vi "Translator.File.ReadGui.vi"(6 "~Do not save font? (F)":bool, 8 "~error in":errorcluster, 10 "~Language in use":string="English", 11 "~Translation folder":path=path "D:/PL_0125_Sapphire_Automation_branches/SOFTWARE_v1.1-Translation/settings") -> (0 "~error out":errorcluster, 1 "~restart?":bool, 2 "~font name":string)   [LabVIEW 2013]
uses:
  <vilib>/Utility/miscctls.llb/LVBoundsTypeDef.ctl
  Translator.Global.vi
  Config/Config.Global.vi
panel:
  out "~progressbar2":i32(slide) scale=-1.1..10.0
  out "~progressbar1":i32(slide) scale=0.0..17.0
  out "Message":string
  out "~flag":picture
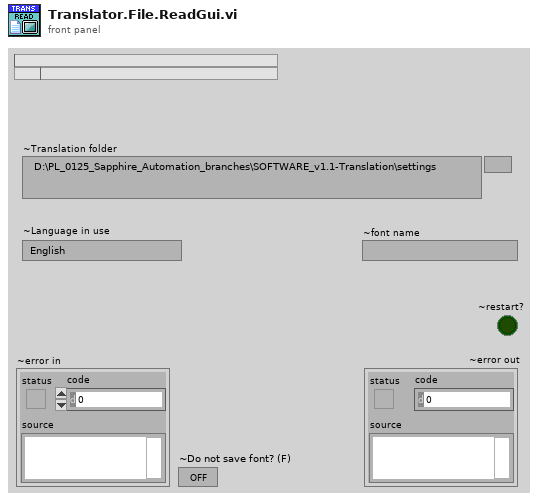
[diagram p1: front panel]
types:
  T1 = typedef "LVBoundsTypeDef.ctl" = cluster{"Width":u32, "Height":u32}
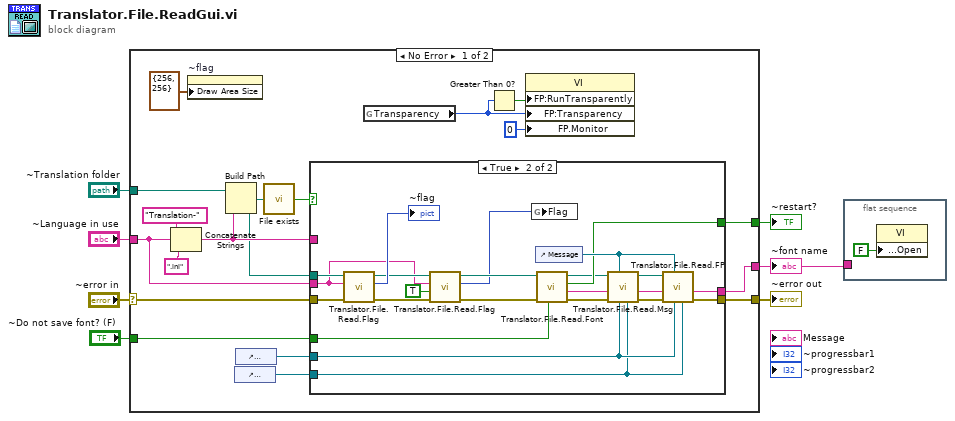
[diagram p0: block diagram]
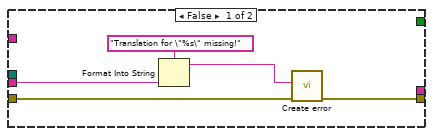
[diagram p2: hidden frame]
diagram:
  n1 = case shown="No Error" "~error in" {
    selector: "~error in" -> [w16 w48]
    tunnel: "~Translation folder" -> [w11 _]
    tunnel: [w23 w48] -> w4
    tunnel: "~Language in use" -> [w15 _]
    tunnel: [w13 _] -> w3
    tunnel: [w18 _] -> w2
    tunnel: "~Do not save font? (F)" -> [w12 _]
    frame No Error {
      n2 = Concatenate Strings("Translation-" ("string"), w15, ".ini" ("string")) -> (w22:string)
      n3 = property on="~flag" class="Pict"("Draw Area Size"=T1 {"Width"=256, "Height"=256}) -> ()  [unwired: 2 in, 2 out]
      n4 = Build Path(base path=w11, name or relative path=w22) -> (appended path=w17:path)
      n5 = control-ref of="~progressbar2"() -> (w19:refnum<vi>)
      n6 = control-ref of="~progressbar1"() -> (w20:refnum<vi>)
      n7 = call "File exists.vi"("file path"=w17) -> ("exists?"=w21:bool)  [unwired: 4 in]
      n8 = case shown="True" w21 {
        tunnel: w16 -> [w29 w39]
        tunnel: [_ w47] -> w13
        tunnel: [w30 w46] -> w23
        tunnel: w17 -> [_ w37]
        tunnel: w22 -> [_ _]
        tunnel: w20 -> [_ w45]
        tunnel: w19 -> [_ w44]
        tunnel: [_ w42] -> w18
        tunnel: w15 -> [w26 w34]
        tunnel: w12 -> [_ w31]
        frame False {
          n9 = Format Into String(format string="Translation for \"%s\" missing!", w26) -> (resulting string=w27:string)  [unwired: 2 in, 1 out]
          n10 = call "Create error.vi"("error in"=w29, "explanation"=w27) -> ("error out"=w30:errorcluster)  [unwired: 9 in]
        }
        frame True {
          n11 = call "Translator.File.Read.Flag.vi"("error in"=w39, "Language in use"=w34, "Translation file"=w37) -> ("error out"=w36:errorcluster, "~flag"=→"~flag":picture)  [unwired: 6 in, 1 out]
          n12 = call "Translator.File.Read.Flag.vi"("error in"=w36, "miniature (F)"=TRUE, "Language in use"=w34, "Translation file"=w37) -> ("error out"=w35:errorcluster, "~flag"=w32:picture)  [unwired: 5 in, 1 out]
          n13 = global write "Translator.Global.vi" "Flag"(w32) -> ()
          n14 = control-ref of="Message"() -> (w43:refnum<vi>)
          n15 = call "Translator.File.Read.Font.vi"("Do not save font? (F)"=w31, "error in"=w35, "Translation file"=w37) -> ("error out"=w41:errorcluster, "font name"=w47:string, "restart required?"=w42:bool)  [unwired: 6 in]
          n16 = call "Translator.File.Read.Msg.vi"("progressbar2"=w44, "progressbar1"=w45, "Message"=w43, "error in"=w41, "Translation folder"=w37) -> ("error out"=w40:errorcluster)  [unwired: 6 in]
          n17 = call "Translator.File.Read.FP.vi"("progressbar2"=w44, "progressbar1"=w45, "Message"=w43, "error in"=w40, "font name"=w47, "Translation file"=w37) -> ("error out"=w46:errorcluster)  [unwired: 5 in]
        }
      }
      n18 = global read "Config.Global.vi" "Transparency"() -> (w8:u8)
      n19 = Greater Than 0?(x=w8) -> (x > 0?=w10:bool)
      n20 = property class="VI"("FP:RunTransparently"=w10, "FP:Transparency"=w8, "FP.Monitor"=u16 0 ("Front Panel Window:Monitor")) -> ()  [unwired: 2 in, 2 out]
    }
    frame Error {
    }
  }
  "~error out" <- w4
  "~font name" <- w3
  "~restart?" <- w2
  n21 = flat-sequence {
    tunnel: w3 -> [_]
    frame #0 {
      n22 = property class="VI"("Front Panel.Open"=FALSE ("Front Panel Window:Open")) -> ()  [unwired: 2 in, 2 out]
    }
  }
